vi "Day 21-Recursive.vi"(10 "Map":map{u64, u64}(c390), 11 "State":T1) -> (2 "Player 2 Win Count out":u64, 3 "Player 1 Win Count out":u64)   [LabVIEW 2021]
uses:
  Day 21-Turn Cluster.ctl
  Day 21-Player Turn.ctl
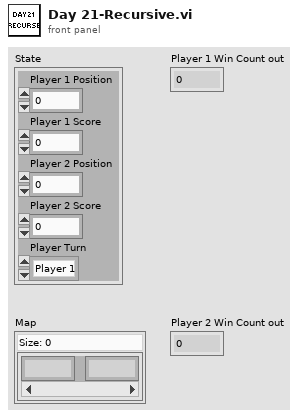
[diagram p1: front panel]
types:
  T1 = typedef "Day 21-Turn Cluster.ctl" = cluster{"Player 1 Position":u64, "Player 1 Score":u64, "Player 2 Position":u64, "Player 2 Score":u64, "Player Turn":T2}
  T2 = typedef "Day 21-Player Turn.ctl" = enum16{"Player 1", "Player 2"}
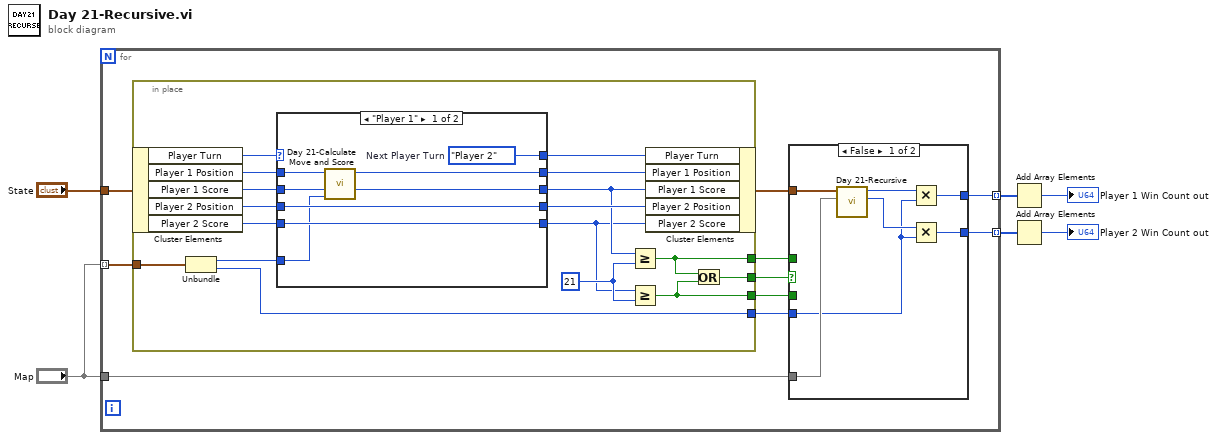
[diagram p0: block diagram]
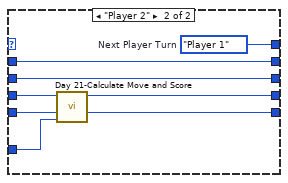
[diagram p2: hidden frame]
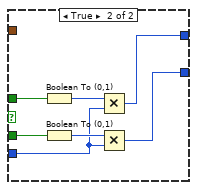
[diagram p3: hidden frame]
diagram:
  n1 = for {
    tunnel: "State" -> [w16]
    tunnel: [w11] -> w1 mode=indexing
    tunnel: [w10] -> w3 mode=indexing
    tunnel: "Map" -> [w9]
    tunnel: "Map" -> [w8] mode=indexing
    n2 = in-place {
      in-place-border: [w25] -> w13
      in-place-border: [w23] -> w14
      in-place-border: [w22] -> w15
      in-place-border: w8 -> [w21]
      in-place-border: [w19] -> w7
      w26 = u64 21
      n3 = in-place-cluster #1(w16) -> ("Player Turn"=w33:T2, "Player 1 Position"=w32:u64, "Player 1 Score"=w31:u64, "Player 2 Position"=w29:u64, "Player 2 Score"=w27:u64)
      n4 = Unbundle(w21) -> (w20:u64, "value"=w19:u64)
      n5 = case shown="\"Player 1\"" w33 {
        tunnel: w32 -> [w41 w43]
        tunnel: w29 -> [w40 w48]
        tunnel: w20 -> [w36 w44]
        tunnel: w31 -> [w35 w42]
        tunnel: [w34 w42] -> w18
        tunnel: [w38 w43] -> w30
        tunnel: [w40 w47] -> w28
        tunnel: [w39 w45] -> w17
        tunnel: w27 -> [w39 w46]
        tunnel: [w37 w49] -> w24
        frame "Player 1" {
          w37 = Day_21-Player_Turn."Player 2"  # Next Player Turn
          n6 = call "Day 21-Calculate Move and Score.vi"("Dice Roll Sum"=w36, "Score in"=w35, "Position in"=w41) -> ("Score out"=w34:u64, "Position out"=w38:u64)  [unwired: 7 in]
        }
        frame "Player 2" {
          w49 = Day_21-Player_Turn."Player 1"  # Next Player Turn
          n7 = call "Day 21-Calculate Move and Score.vi"("Dice Roll Sum"=w44, "Score in"=w46, "Position in"=w48) -> ("Score out"=w45:u64, "Position out"=w47:u64)  [unwired: 7 in]
        }
      }
      n8 = Greater Or Equal?(x=w18, y=w26) -> (x >= y?=w23:bool)
      n9 = Greater Or Equal?(x=w17, y=w26) -> (x >= y?=w22:bool)
      n10 = in-place-cluster #1("Player Turn"=w24, "Player 1 Position"=w30, "Player 1 Score"=w18, "Player 2 Position"=w28, "Player 2 Score"=w17) -> (w12:T1)
      n11 = Or(x=w23, y=w22) -> (x .or. y?=w25:bool)
    }
    n12 = case shown="False" w13 {
      tunnel: w12 -> [w56 _]
      tunnel: w14 -> [_ w63]
      tunnel: [w51 w58] -> w10
      tunnel: w15 -> [_ w59]
      tunnel: [w50 w57] -> w11
      tunnel: w9 -> [w55 _]
      tunnel: w7 -> [w52 w60]
      frame False {
        n13 = call "Day 21-Recursive.vi"("Map"=w55, "State"=w56) -> ("Player 2 Win Count out"=w53:u64, "Player 1 Win Count out"=w54:u64)  [unwired: 8 in]
        n14 = Multiply(x=w54, y=w52) -> (x*y=w51:u64)
        n15 = Multiply(x=w53, y=w52) -> (x*y=w50:u64)
      }
      frame True {
        n16 = Boolean To (0,1)(Boolean=w63) -> (0, 1=w62:i16)
        n17 = Boolean To (0,1)(Boolean=w59) -> (0, 1=w61:i16)
        n18 = Multiply(x=w62, y=w60) -> (x*y=w58:u64)
        n19 = Multiply(x=w61, y=w60) -> (x*y=w57:u64)
      }
    }
  }
  n20 = Add Array Elements(numeric array=w3) -> (sum=→"Player 1 Win Count out":u64)
  n21 = Add Array Elements(numeric array=w1) -> (sum=→"Player 2 Win Count out":u64)
